vi "CCD-PDA_ExposureTime.vi"(1 "Current Detector":T1, 4 "CCD Parameters":T2={"Exposure Time (s)"=0.2, "Offset"=0.0, "BkgrdCrct"=FALSE, "Shutter"=FALSE, "Mode"=enum."Regular", "Repetition"=4, "dt or s"=0.0} {"dt or s" format="%#.6f"; "Repetition" min=1; "Offset" format="%#.2f"; "Exposure Time (s)" min=0.02 max=6000.0 format="%#.2f"}) -> (0 "Exposure Time (s)":dbl)   [LabVIEW 2024]
doc: "This is the controlling VI for CCD exposures.\nIt calls the right CCD subVIs if the \"Current Experiment Status\" Exposure status is \"OK\".\nIt will also set the \"Current Experiment Status\" Exposure status \nfrom \"OK\" to \"Busy\" to \"Done\" ."
uses:
  Globals and TypeDefs/Type Definitions.llb/CCDParameter.ctt
  Globals and TypeDefs/Type Definitions.llb/ListOfDetectors.ctt
  Globals and TypeDefs/gDetector.vi
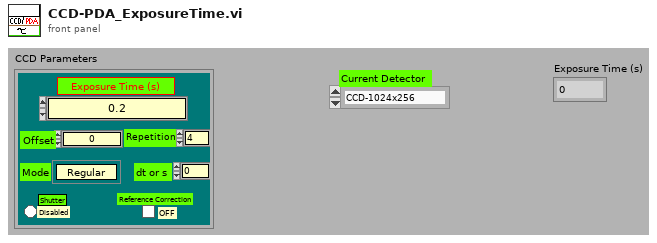
[diagram p1: front panel]
types:
  T1 = typedef "ListOfDetectors.ctt" = enum8{"CCD-1024x256", "InGaAs PDA-1024x1", "CCD-1340x400", "Ge Single Channel", "Si Single Channel", "PMT Single Channel"}
  T2 = typedef "CCDParameter.ctt" = cluster{"Exposure Time (s)":dbl, "Offset":dbl, "BkgrdCrct":bool, "Shutter":bool, "Mode":enum8{"Regular", "OverExp Cor", "SpikeRemove", "ForCalibration"}, "Repetition":u16, "dt or s":dbl}
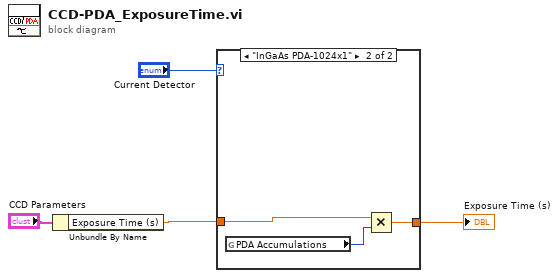
[diagram p0: block diagram]
diagram:
  n1 = Unbundle By Name("CCD Parameters") -> ("Exposure Time (s)"=w2:dbl)
  n2 = case shown="\"InGaAs PDA-1024x1\"" "Current Detector" {
    tunnel: [w5 w7] -> w1
    tunnel: w2 -> [w5 w8]
    frame "CCD-1024x256", Default {
    }
    frame "InGaAs PDA-1024x1" {
      n3 = global read "gDetector.vi" "PDA Accumulations"() -> (w6:i32)
      n4 = Multiply(x=w8, y=w6) -> (x*y=w7:dbl)
    }
  }
  "Exposure Time (s)" <- w1
